vi "setWavelength.vi"(8 "error in (no error)":errorcluster, 9 "Monochromator in":refnum<class "Monochromator.lvclass">, 10 "wavelength":T1, 11 "MonoState in":refnum<class "MonoState.lvclass">) -> (0 "error out":errorcluster, 1 "Monochromator out":refnum<class "Monochromator.lvclass">, 3 "MonoState out":refnum<class "MonoState.lvclass">)   [LabVIEW 2016, in "MonoState.lvclass"]
uses:
  MonoState.lvclass
  Typedefs/wavelength.ctl
  Monochromator/Monochromator.lvclass
  Typedefs/AckType.ctl
  Monochromator/Monochromator.lvclass/Monochromator.ctl
  MonoCommunicator/MonoCommunicator.lvclass
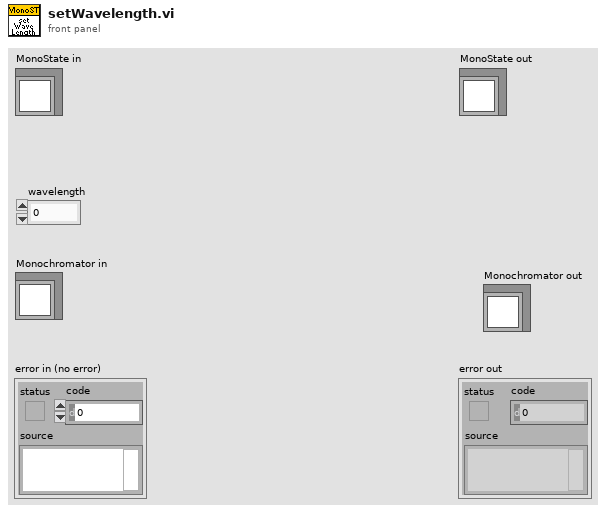
[diagram p1: front panel]
types:
  T1 = typedef "wavelength.ctl" = dbl
  T2 = typedef "AckType.ctl" = enum16{"OK", "OutOfRange", "Unknown", "Busy", "Rejected"}
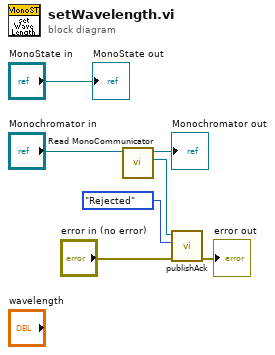
[diagram p0: block diagram]
diagram:
  n1 = call "Read MonoCommunicator.vi"("Monochromator in"="Monochromator in") -> ("MonoCommunicator.lvclass"=w2:refnum<class "MonoCommunicator.lvclass">, "Monochromator out"=→"Monochromator out":refnum<class "Monochromator.lvclass">)  [unwired: 8 in, 1 out]
  n2 = call "publishAck.vi"("error in (no error)"="error in (no error)", "AckType"=AckType."Rejected", "MonoCommunicator in"=w2) -> ("error out"=→"error out":errorcluster)  [unwired: 7 in, 1 out]
  "MonoState out" <- "MonoState in"
